vi "BRig_dataCurrent_DAB_T_Reward_L.vi"() -> (2 "output_DAB_T_Reward_L":i32)   [LabVIEW 2014]
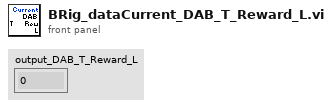
[diagram p1: front panel]
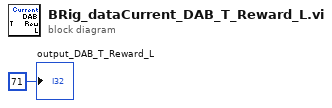
[diagram p0: block diagram]
diagram:
  "output_DAB_T_Reward_L" <- 71 ("output_iBlock")
